vi "SetXScale.vi"(0 "reference":refnum<vi>, 1 "Start":dbl, 2 "End":dbl, 3 "error in":errorcluster, 4 "Step":dbl) -> (5 "error out":errorcluster)   [LabVIEW 2011]
doc: "Sets the value of a front-panel control.\nParameters:\nany:ctrl, Ctrl.\nany:value, new value for control/indicator.\nErrors:\nNot a Ctrl.\nData type of value does not match data type of control/indicator.\nData type of control/indicator not supported."
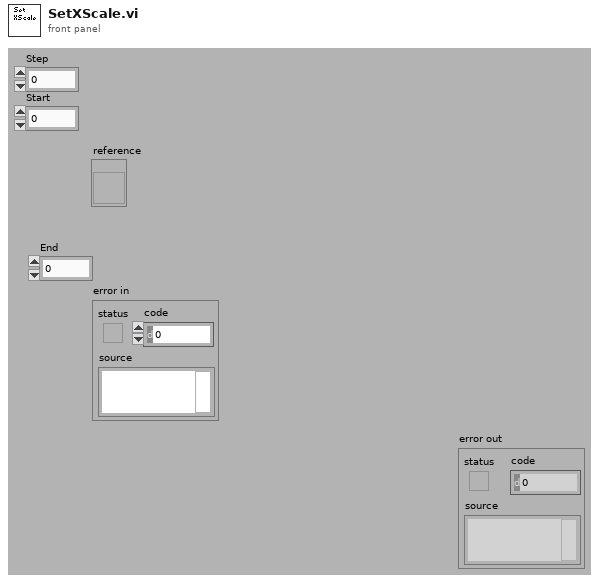
[diagram p1: front panel]
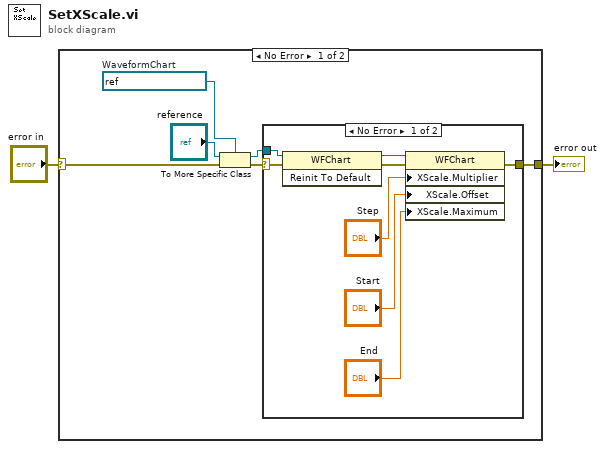
[diagram p0: block diagram]
diagram:
  n1 = case shown="No Error" "error in" {
    selector: "error in" -> [w5 w18]
    tunnel: [w8 w18] -> w2
    frame No Error {
      w6 = refnum<vi> refnum  # WaveformChart
      n2 = To More Specific Class(target class=w6, reference="reference", error in=w5) -> (specific class reference=w3:refnum<vi>, error out=w4:errorcluster)
      n3 = case shown="No Error" w4 {
        selector: w4 -> [w10 w17]
        tunnel: [w13 w17] -> w8
        tunnel: w3 -> [w12 _]
        frame No Error {
          n4 = invoke class="WFChart" method="Reinit To Default"(reference=w12, error in=w10) -> (reference out=w11:refnum<vi>, error out=w9:errorcluster)  [unwired: 1 in, 1 out]
          n5 = property on="Property Node" class="WFChart"(reference=w11, error in=w9, "XScale.Multiplier"="Step", "XScale.Offset"="Start", "XScale.Maximum"="End") -> (error out=w13:errorcluster)  [unwired: 1 out]
        }
        frame Error {
        }
      }
    }
    frame Error {
    }
  }
  "error out" <- w2
